vi "ActiveObjects_DynamicEvents_ProcessRepository_Native.vi"(0 "reference in":refnum<class>, 1 "Action(ReadRepository)":T1(ring), 5 "error in (no error)":errorcluster) -> (7 "QueueFromProcess":refnum<queue>, 9 "ProcessViRef":refnum<vi>, 11 "ProcessSyncQueue":refnum<queue>, 13 "EventFromProcess":refnum<user-event>, 14 "reference out":refnum<class>, 15 "EventsToProcess":refnum<user-event>, 17 "ProcessAlreadyStarted":bool, 19 "error out":errorcluster)   [LabVIEW 2010]
uses:
  ActiveObjects_DynamicEvents_Process.ctl
panel:
  # "Use this indicator for sending messages to the Process VI"
  # "These indicators are used by the process VIs"
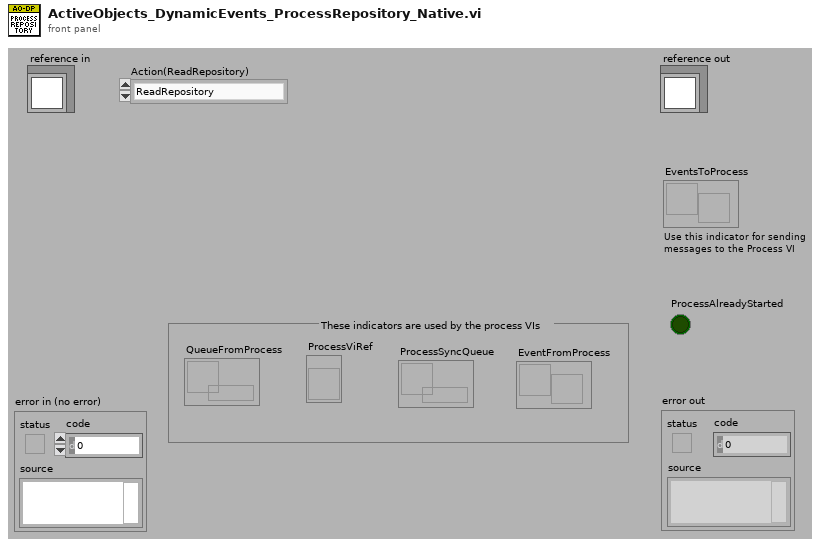
[diagram p1: front panel]
types:
  T1 = enum16{"ReadRepository", "CreateNew", "CreateOrLookUpExisting"}
  T2 = typedef "ActiveObjects_DynamicEvents_Process.ctl" = cluster{"EventsToProcess":refnum<user-event>, "EventFromProcess":refnum<user-event>, "ProcessSyncQueue":refnum<queue>, "ProcessViRef":refnum<vi>, "QueueFromProcess":refnum<queue>}
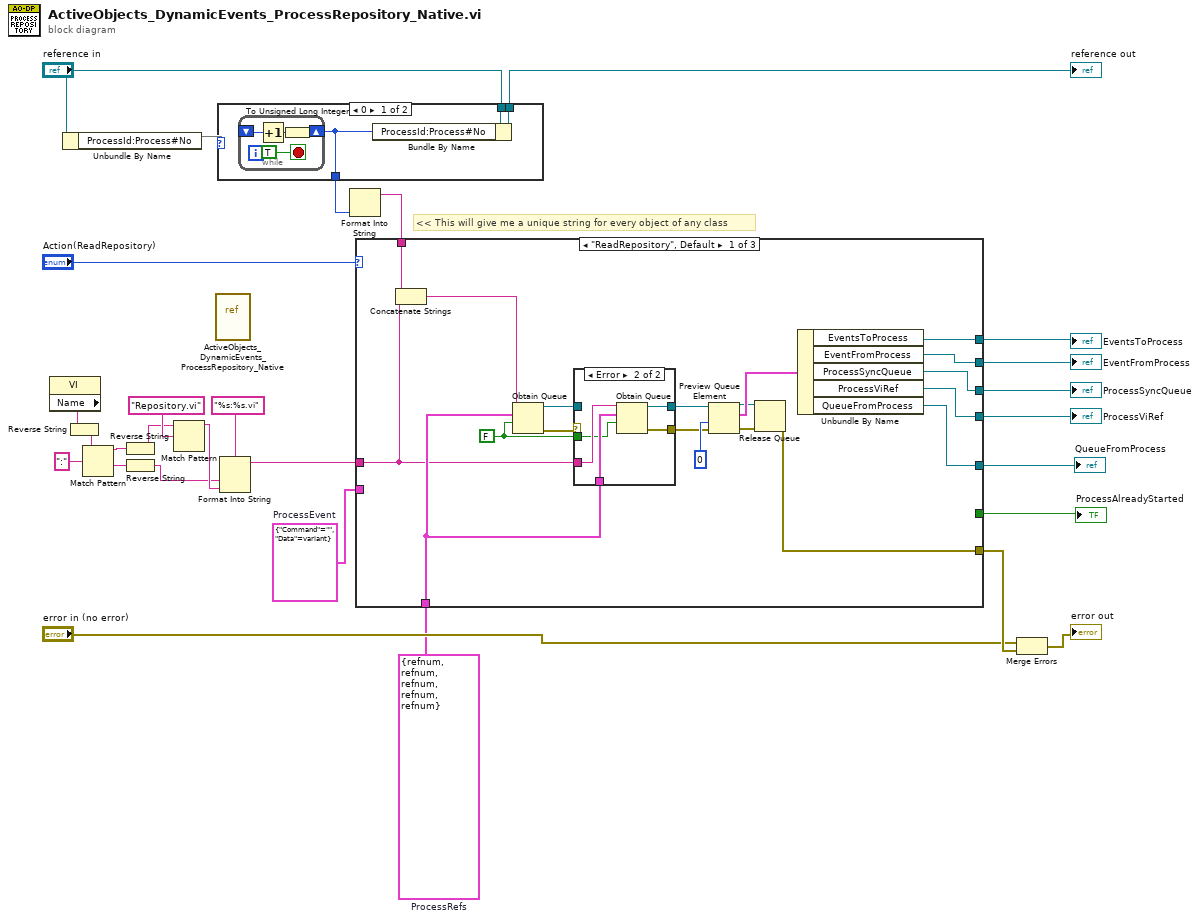
[diagram p0: block diagram]
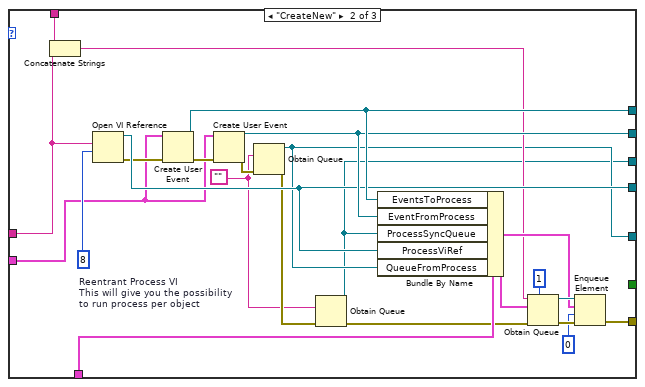
[diagram p4: hidden frame]
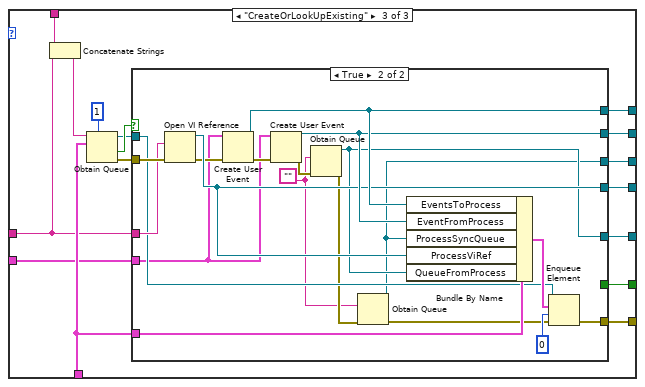
[diagram p5: hidden frame]
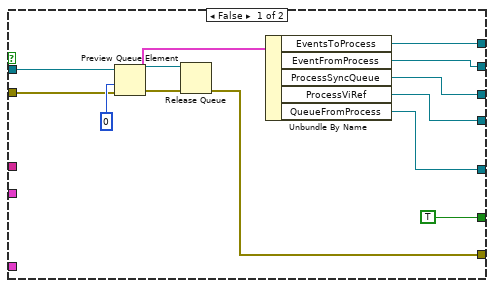
[diagram p6: hidden frame]
diagram:
  w1 = T2 {"EventsToProcess"=refnum, "EventFromProcess"=refnum, "ProcessSyncQueue"=refnum, "ProcessViRef"=refnum, "QueueFromProcess"=refnum}  # ProcessRefs
  w3 = cluster{"Command":string, "Data":variant} {"Command"="", "Data"=variant}  # ProcessEvent
  # "<< This will give me a unique string for every object of any class"
  n1 = property class="VI"() -> ("Name"=w13:string)  [unwired: 2 in, 2 out]
  n2 = Unbundle By Name("reference in") -> ("ProcessId:Process#No"=w7)
  n3 = Reverse String(1:w13) -> (0:w14:string)
  n4 = Match Pattern(string=w14, regular expression=":") -> (before substring=w18:string, after substring=w15:string)  [unwired: 1 in, 2 out]
  n5 = Reverse String(1:w18) -> (0:w19:string)
  n6 = Reverse String(1:w15) -> (0:w17:string)
  n7 = Match Pattern(string=w19, regular expression="Repository.vi") -> (before substring=w21:string)  [unwired: 1 in, 3 out]
  n8 = vi-ref "ActiveObjects_DynamicEvents_ProcessRepository_Native.vi"() -> ()  [unwired: 1 out]
  n9 = case shown="0" w7 {
    selector: w7 -> [_ w37]
    tunnel: [w29 w37] -> w8
    tunnel: "reference in" -> [w31 w36]
    tunnel: [w30 w36] -> w5
    frame 0 {
      n10 = while {
        shift-right: [w32] -> w29
        shift-left: _ -> [w34]
        stop <- TRUE stop-if-true
        n11 = Increment(x=w34) -> (x+1=w33:u32)
        n12 = To Unsigned Long Integer(number=w33) -> (unsigned 32bit integer=w32:u32)
      }
      n13 = Bundle By Name(cluster=w31, "ProcessId:Process#No"=w29) -> (w30:refnum<class>)
    }
    frame Default {
    }
  }
  "reference out" <- w5
  n14 = Format Into String(format string="%s:%s.vi", w17, w21) -> (resulting string=w11:string)  [unwired: 2 in, 1 out]
  n15 = Format Into String(w8) -> (resulting string=w4:string)  [unwired: 3 in, 1 out]
  n16 = case shown="\"ReadRepository\", Default" "Action(ReadRepository)" {
    tunnel: [w52 w64 w100] -> w27
    tunnel: [w54 w86 w102] -> w25
    tunnel: [w53 w85 w101] -> w26
    tunnel: [w55 w84 w99] -> w24
    tunnel: w1 -> [w47 w74 w95]
    tunnel: w4 -> [w45 w73 w91]
    tunnel: [w38 w83 w98] -> w22
    tunnel: w11 -> [w44 w71 w90]
    tunnel: [_ _ w93] -> w10
    tunnel: w3 -> [_ w70 w88]
    tunnel: [w42 w68 w87] -> w2
    frame "ReadRepository", Default {
      w46 = FALSE ("create if not found? (T)")
      n17 = Concatenate Strings(w45, w44) -> (w43:string)
      n18 = Obtain Queue(name (unnamed)=w43, element data type=w47, create if not found? (T)=w46) -> (queue out=w49:refnum<queue>, error out=w51:errorcluster)  [unwired: 2 in, 1 out]
      n19 = case shown="Error" w51 {
        selector: w51 -> [w58 _]
        tunnel: [w58 w60] -> w50
        tunnel: w49 -> [w57 _]
        tunnel: [w57 w61] -> w48
        tunnel: w47 -> [_ w63]
        tunnel: w44 -> [_ w62]
        tunnel: w46 -> [_ w59]
        frame No Error {
        }
        frame Error {
          n20 = Obtain Queue(name (unnamed)=w62, element data type=w63, create if not found? (T)=w59) -> (queue out=w61:refnum<queue>, error out=w60:errorcluster)  [unwired: 2 in, 1 out]
        }
      }
      n21 = Preview Queue Element(queue=w48, timeout in ms (-1)=0, error in (no error)=w50) -> (queue out=w40:refnum<queue>, element=w41:T2, error out=w39:errorcluster)  [unwired: 1 out]
      n22 = Release Queue(queue=w40, error in (no error)=w39) -> (error out=w38:errorcluster)  [unwired: 1 in, 2 out]
      n23 = Unbundle By Name(w41) -> ("EventsToProcess"=w54:refnum<user-event>, "EventFromProcess"=w53:refnum<user-event>, "ProcessSyncQueue"=w52:refnum<queue>, "ProcessViRef"=w55:refnum<vi>, "QueueFromProcess"=w42:refnum<queue>)
    }
    frame "CreateNew" {
      w65 = ""
      w80 = 8  # Reentrant Process VI This will give you the possibility to run process per object
      n24 = Concatenate Strings(w73, w71) -> (w72:string)
      n25 = Open VI Reference(vi path=w71, options=w80) -> (vi reference=w84:refnum<vi>, error out=w81:errorcluster)  [unwired: 4 in]
      n26 = Create User Event(user event datatype=w70, error in=w81) -> (user event=w86:refnum<user-event>, error out=w82:errorcluster)
      n27 = Create User Event(user event datatype=w70, error in=w82) -> (user event=w85:refnum<user-event>, error out=w69:errorcluster)
      n28 = Obtain Queue(element data type=w65, error in (no error)=w69) -> (queue out=w68:refnum<queue>, error out=w67:errorcluster)  [unwired: 3 in, 1 out]
      n29 = Obtain Queue(element data type=w65, error in (no error)=w67) -> (queue out=w64:refnum<queue>, error out=w66:errorcluster)  [unwired: 3 in, 1 out]
      n30 = Bundle By Name(cluster=w74, "EventsToProcess"=w86, "EventFromProcess"=w85, "ProcessSyncQueue"=w64, "ProcessViRef"=w84, "QueueFromProcess"=w68) -> (w77:T2)
      n31 = Obtain Queue(max queue size (-1, unlimited)=1, name (unnamed)=w72, element data type=w77, error in (no error)=w66) -> (queue out=w79:refnum<queue>, error out=w78:errorcluster)  [unwired: 1 in, 1 out]
      n32 = Enqueue Element(queue=w79, element=w77, timeout in ms (-1)=0, error in (no error)=w78) -> (error out=w83:errorcluster)  [unwired: 2 out]
    }
    frame "CreateOrLookUpExisting" {
      n33 = Concatenate Strings(w91, w90) -> (w89:string)
      n34 = Obtain Queue(max queue size (-1, unlimited)=1, name (unnamed)=w89, element data type=w95) -> (queue out=w96:refnum<queue>, created new?=w97:bool, error out=w94:errorcluster)  [unwired: 2 in]
      n35 = case shown="True" w97 {
        tunnel: [w115 w134] -> w102
        tunnel: [w114 w133] -> w101
        tunnel: [w113 w117] -> w100
        tunnel: [w112 w132] -> w99
        tunnel: [w103 w131] -> w98
        tunnel: w95 -> [_ w130]
        tunnel: w94 -> [w109 w125]
        tunnel: w90 -> [_ w124]
        tunnel: w96 -> [w110 w123]
        tunnel: [TRUE _] -> w93
        tunnel: w88 -> [_ w122]
        tunnel: [w106 w120] -> w87
        frame False {
          n36 = Preview Queue Element(queue=w110, timeout in ms (-1)=0, error in (no error)=w109) -> (queue out=w105:refnum<queue>, element=w108:T2, error out=w104:errorcluster)  [unwired: 1 out]
          n37 = Release Queue(queue=w105, error in (no error)=w104) -> (error out=w103:errorcluster)  [unwired: 1 in, 2 out]
          n38 = Unbundle By Name(w108) -> ("EventsToProcess"=w115:refnum<user-event>, "EventFromProcess"=w114:refnum<user-event>, "ProcessSyncQueue"=w113:refnum<queue>, "ProcessViRef"=w112:refnum<vi>, "QueueFromProcess"=w106:refnum<queue>)
        }
        frame True {
          w118 = ""
          n39 = Open VI Reference(vi path=w124, error in (no error)=w125) -> (vi reference=w132:refnum<vi>, error out=w128:errorcluster)  [unwired: 4 in]
          n40 = Create User Event(user event datatype=w122, error in=w128) -> (user event=w134:refnum<user-event>, error out=w129:errorcluster)
          n41 = Create User Event(user event datatype=w122, error in=w129) -> (user event=w133:refnum<user-event>, error out=w121:errorcluster)
          n42 = Obtain Queue(element data type=w118, error in (no error)=w121) -> (queue out=w120:refnum<queue>, error out=w119:errorcluster)  [unwired: 3 in, 1 out]
          n43 = Obtain Queue(element data type=w118, error in (no error)=w119) -> (queue out=w117:refnum<queue>, error out=w116:errorcluster)  [unwired: 3 in, 1 out]
          n44 = Bundle By Name(cluster=w130, "EventsToProcess"=w134, "EventFromProcess"=w133, "ProcessSyncQueue"=w117, "ProcessViRef"=w132, "QueueFromProcess"=w120) -> (w127:T2)
          n45 = Enqueue Element(queue=w123, element=w127, timeout in ms (-1)=0, error in (no error)=w116) -> (error out=w131:errorcluster)  [unwired: 2 out]
        }
      }
    }
  }
  "ProcessSyncQueue" <- w27
  "EventsToProcess" <- w25
  "EventFromProcess" <- w26
  "ProcessViRef" <- w24
  "ProcessAlreadyStarted" <- w10
  "QueueFromProcess" <- w2
  n46 = Merge Errors("error in (no error)", w22) -> (→"error out":errorcluster)
